vi "Add Pattern Script Header.vi"(8 "error in (no error)":errorcluster, 9 "Pattern Script Frame in":string, 10 "Pattern Name":string, 11 "SPI 3W Pattern Creator in":refnum<class "SPI 3W Pattern Creator.lvclass">) -> (0 "error out":errorcluster, 2 "Pattern Script All out":string, 3 "SPI 3W Pattern Creator out":refnum<class "SPI 3W Pattern Creator.lvclass">)   [LabVIEW 2018, in "SPI 3W Pattern Creator.lvlib" / "SPI 3W Pattern Creator.lvclass"]
uses:
  SPI 3W Pattern Creator.lvclass
  Interfaces/Protocol Interface.lvlibp/Interfaces/Protocol Interface/Pin State.ctl
  Interfaces/Protocol Interface.lvlibp/Interfaces/Protocol Interface/Protocol Interface.lvclass
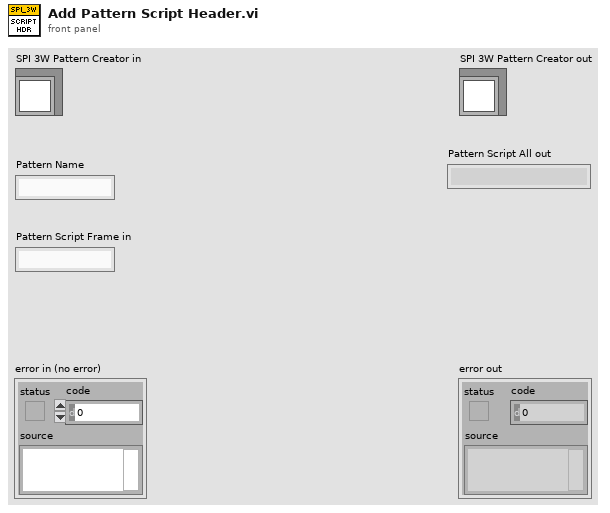
[diagram p1: front panel]
types:
  T1 = typedef "Protocol Interface.lvlibp/Protocol Interface.lvclass/Pin State.ctl" = enum16{"0", "1", "L", "H", "X", "V", "D", "M"}
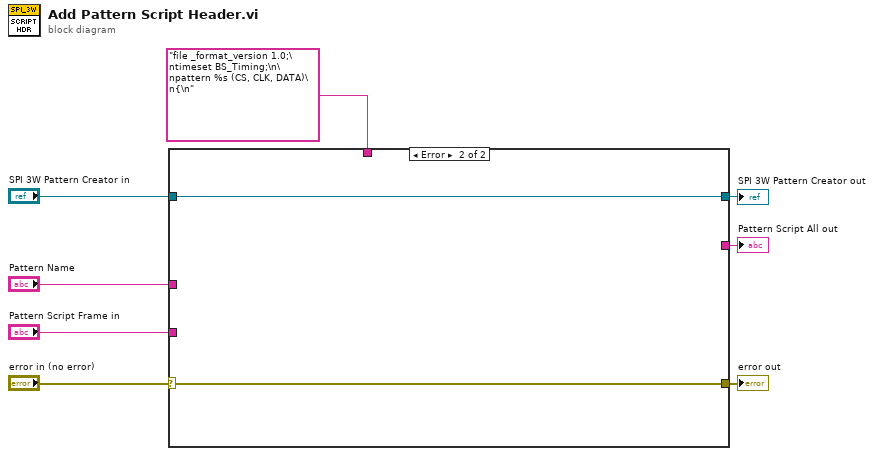
[diagram p0: block diagram]
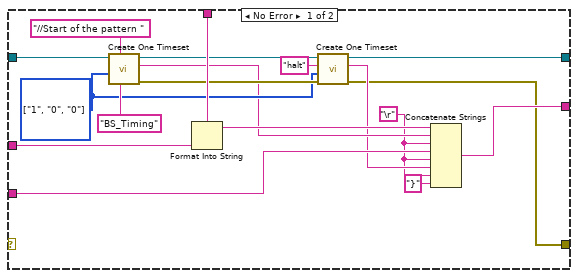
[diagram p2: hidden frame]
diagram:
  n1 = case shown="Error" "error in (no error)" {
    selector: "error in (no error)" -> [_ w27]
    tunnel: "Pattern Name" -> [w26 _]
    tunnel: "file _format_version 1.0;\ntimeset BS_Timing;\n\npattern %s (CS, CLK, DATA)\n{\n" -> [w25 _]
    tunnel: "SPI 3W Pattern Creator in" -> [w24 w28]
    tunnel: "Pattern Script Frame in" -> [w14 _]
    tunnel: [w17 w28] -> w3
    tunnel: [w10 _] -> w2
    tunnel: [w9 w27] -> w1
    frame No Error {
      w12 = "\r"
      w18 = T1[] [enum."1", enum."0", enum."0"] items=["0", "1", "L", "H", "X", "V", "D", "M"] ("PinStates")
      n2 = call-dynamic "Create One Timeset.vi"("Timeset Name"="BS_Timing", "Notes"="//Start of the pattern ", "PinStates"=w18, "SPI 3W Pattern Creator in"=w24) -> ("error out"=w20:errorcluster, "String  out"=w15:string, "SPI 3W Pattern Creator out"=w21:refnum<class "SPI 3W Pattern Creator.lvclass">)  [unwired: 5 in]
      n3 = Format Into String(format string=w25, w26) -> (resulting string=w16:string)  [unwired: 2 in, 1 out]
      n4 = call-dynamic "Create One Timeset.vi"("error in (no error)"=w20, "PinStates"=w18, "OpCode"="halt", "SPI 3W Pattern Creator in"=w21) -> ("error out"=w9:errorcluster, "String  out"=w13:string, "SPI 3W Pattern Creator out"=w17:refnum<class "SPI 3W Pattern Creator.lvclass">)  [unwired: 5 in]
      n5 = Concatenate Strings(w16, w15, w12, w14, w12, w13, w12, "}" ("string")) -> (w10:string)
    }
    frame Error {
    }
  }
  "error out" <- w1
  "SPI 3W Pattern Creator out" <- w3
  "Pattern Script All out" <- w2
